vi "AcquisitionInterface.vi"() -> ()   [LabVIEW 2018]
uses:
  <vilib>/Analysis/NI_AAL_SigProc.lvlib
panel:
  out "?":string
  in  "Threshold":dbl
  out "Heart Rate (BPM)":dbl
  out "ECG pós 1º filtro":waveform(dbl)(graph)
  out "ECG pós 2º filtro":waveform(dbl)(graph)
  out "Raw ECG":dynamicdata(graph)
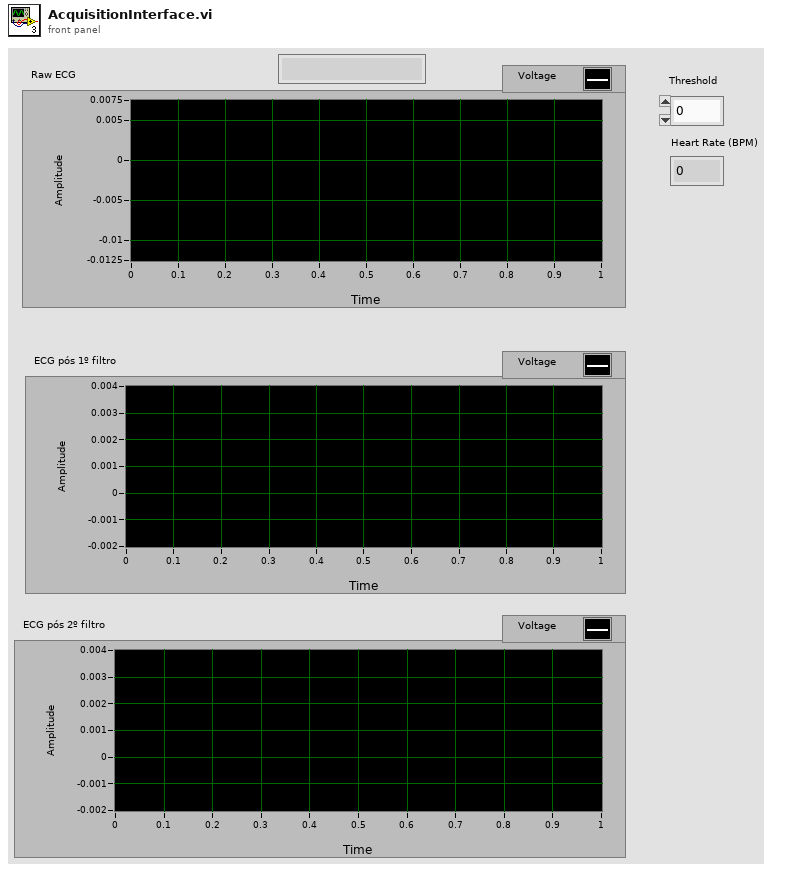
[diagram p1: front panel]
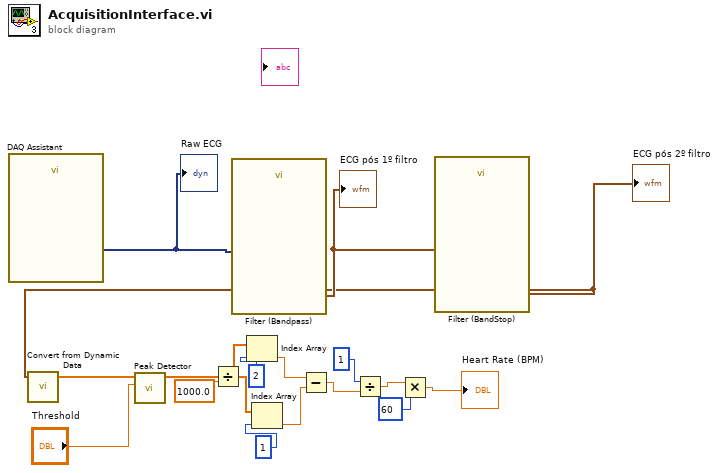
[diagram p0: block diagram]
diagram:
  n1 = call "DAQ Assistant"() -> ("data"=w2:dynamicdata)  [unwired: 17 in, 2 out]
  "Raw ECG" <- w2
  n2 = call "Filter (Bandpass)"("input signal"=w2) -> ("filtered data"=w17:waveform(dbl))  [unwired: 17 in, 1 out]
  "ECG pós 1º filtro" <- w17
  n3 = call "Filter (BandStop)"("input signal"=w17) -> ("filtered data"=w3:waveform(dbl))  [unwired: 17 in, 1 out]
  "ECG pós 2º filtro" <- w3
  n4 = call "Convert from Dynamic Data"("Dynamic Data Type"=w3) -> ("Array"=w16:dbl[])  [unwired: 3 in]
  n5 = call <vilib>:"Peak Detector.vi"("threshold"="Threshold", "X"=w16) -> ("Locations"=w15:dbl[])  [unwired: 5 in, 4 out]
  n6 = Divide(x=w15, y=1000.0) -> (x/y=w4:dbl[])
  n7 = Index Array(array=w4, index=2) -> (element=w11:dbl)
  n8 = Index Array(array=w4, index=1) -> (element=w10:dbl)
  n9 = Subtract(x=w11, y=w10) -> (x-y=w9:dbl)
  n10 = Divide(x=1, y=w9) -> (x/y=w7:dbl)
  n11 = Multiply(x=w7, y=60) -> (x*y=→"Heart Rate (BPM)":dbl)
